vi "lvstyx_open.vi"(8 "error in (no error)":errorcluster, 9 "mode":u16(ring)=1 items=["read"=1, "write"=2, "read/write"=3], 10 "path":string, 11 "client ptr":u32) -> (0 "error out":errorcluster, 3 "file ptr":u32)   [LabVIEW 2010, in "lib1299.lvlib"]
uses:
  lib1299.lvlib
  cstyx/win32/cstyx.dll
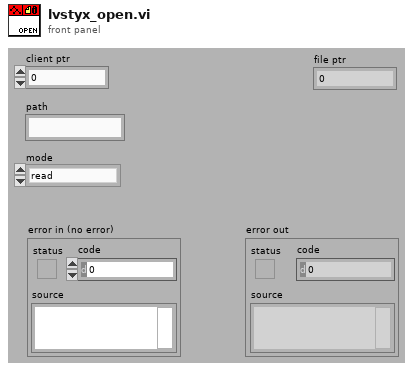
[diagram p1: front panel]
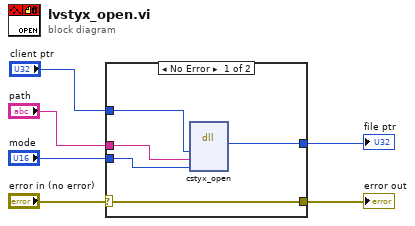
[diagram p0: block diagram]
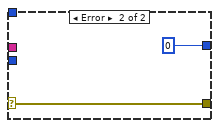
[diagram p2: hidden frame]
diagram:
  n1 = case shown="No Error" "error in (no error)" {
    selector: "error in (no error)" -> [w7 w13]
    tunnel: "path" -> [w11 _]
    tunnel: "mode" -> [w10 _]
    tunnel: "client ptr" -> [w9 _]
    tunnel: [w8 u32 0 ("file")] -> w3
    tunnel: [w7 w13] -> w1
    frame No Error {
      n2 = dll-call lib="C:/work/ads1299evm/lib_1299/Styx/cstyx/win32/cstyx.dll" fn="cstyx_open"("client"=w9, "path"=w11, "mode"=w10) -> ("file"=w8:u32)  [unwired: 6 in, 2 out]
    }
    frame Error {
    }
  }
  "error out" <- w1
  "file ptr" <- w3
